vi "GrowInfo.vi"(1 "XRef":refnum<vi>, 2 "State In":T5) -> (0 "Grow Info":T4)   [LabVIEW 2012, in "OpenG Remove Duplicates from 1 D Array.xnode"]
uses:
  OpenG Remove Duplicates from 1 D Array.xnode
  State.ctl
  <vilib>/XNodeSupport/XNodeBounds.ctl
  <vilib>/XNodeSupport/XNodeInt.ctl
  <vilib>/XNodeSupport/XNodeBool.ctl
  <vilib>/XNodeSupport/NI_XNodeSupport.lvlib
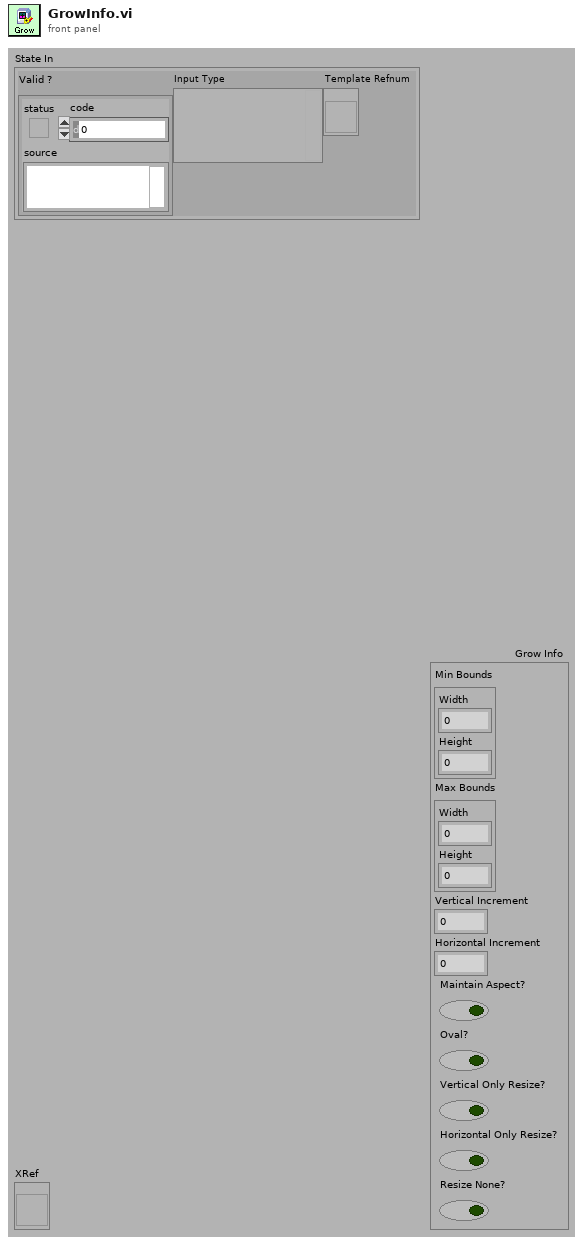
[diagram p1: front panel]
types:
  T1 = typedef "NI_XNodeSupport.lvlib/XNodeBounds.ctl" = cluster{"Width":T2, "Height":T2}
  T2 = typedef "NI_XNodeSupport.lvlib/XNodeInt.ctl" = i32
  T3 = typedef "NI_XNodeSupport.lvlib/XNodeBool.ctl" = bool
  T4 = cluster{"Min Bounds":T1, "Max Bounds":T1, "Vertical Increment":T2, "Horizontal Increment":T2, "Maintain Aspect?":T3, "Oval?":T3, "Vertical Only Resize?":T3, "Horizontal Only Resize?":T3, "Resize None?":T3}
  T5 = typedef "OpenG Remove Duplicates from 1 D Array.xnode/State.ctl" = cluster{"Valid ?":errorcluster, "Input Type":variant, "Template Refnum":refnum<vi>}
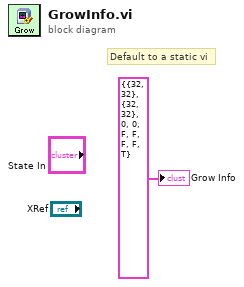
[diagram p0: block diagram]
diagram:
  # "Default to a static vi"
  "Grow Info" <- T4 {"Min Bounds"={"Width"=32, "Height"=32}, "Max Bounds"={"Width"=32, "Height"=32}, "Vertical Increment"=0, "Horizontal Increment"=0, "Maintain Aspect?"=FALSE, "Oval?"=FALSE, "Vertical Only Resize?"=FALSE, "Horizontal Only Resize?"=FALSE, "Resize None?"=TRUE} ("Grow Info")
